vi "Ec. gradul 2.vi"() -> ()   [LabVIEW 2023]
panel:
  out "x2":dbl
  out "x1":dbl
  out "Delta":dbl
  out "Boolean":bool
  in  "c":dbl(slide) scale=-10.0..10.0
  in  "b":dbl(slide) scale=-10.0..10.0
  in  "a":dbl(slide) scale=-10.0..10.0
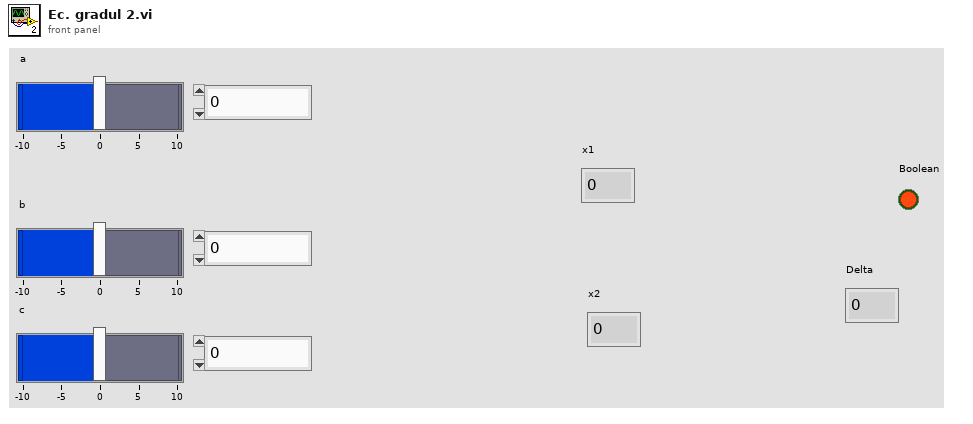
[diagram p1: front panel]
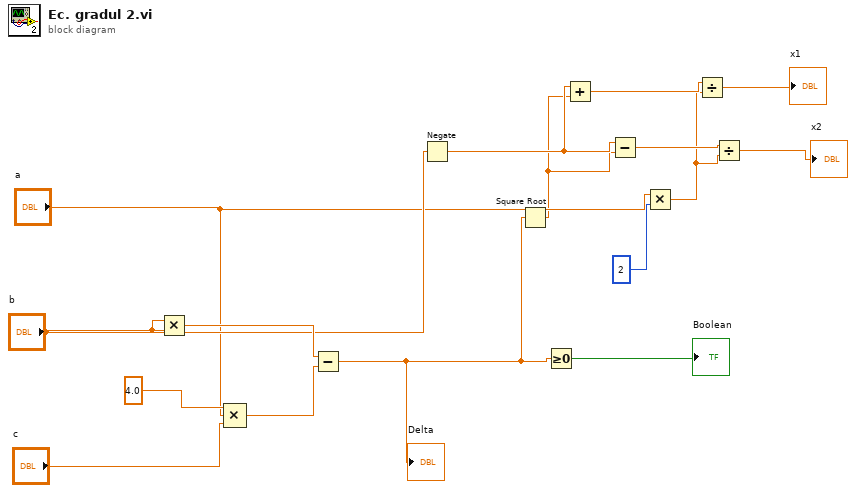
[diagram p0: block diagram]
diagram:
  n1 = Multiply(x="b", y="b") -> (x*y=w14:dbl)
  n2 = Compound Arithmetic op=MULTIPLY(4.0 ("value"), "a", "c") -> (w13:dbl)
  n3 = Subtract(x=w14, y=w13) -> (x-y=w10:dbl)
  "Delta" <- w10
  n4 = Negate(x="b") -> (-x=w5:dbl)
  n5 = Square Root(x=w10) -> (sqrt(x)=w4:dbl)
  n6 = Greater Or Equal To 0?(x=w10) -> (x >= 0?=→"Boolean":bool)
  n7 = Add(x=w5, y=w4) -> (x+y=w9:dbl)
  n8 = Subtract(x=w5, y=w4) -> (x-y=w3:dbl)
  n9 = Multiply(x="a", y=2) -> (x*y=w2:dbl)
  n10 = Divide(x=w9, y=w2) -> (x/y=→"x1":dbl)
  n11 = Divide(x=w3, y=w2) -> (x/y=→"x2":dbl)
